vi "Write JSON Config.vi"(6 "Pretty Print?":bool, 8 "error in (no error)":errorcluster, 11 "ConvertTo_String in":refnum<class "ConvertTo_String.lvclass">) -> (0 "error out":errorcluster, 2 "JSON":string, 3 "ConvertTo_String out":refnum<class "ConvertTo_String.lvclass">)   [LabVIEW 2021, in "ConvertTo_String.lvclass"]
uses:
  ConvertTo_String.lvclass
  C:/Program Files (x86)/National Instruments/LabVIEW 2021/vi.lib/TSA/Abstract Data Classes/Abs_Types/Type/Abs_Type.lvclass
  ConvertTo_String.lvclass/ConvertTo_String.ctl
  <vilib>/JDP Science/JSONtext/Make JSON Array.vi
  <vilib>/JDP Science/JSONtext/Merge into Object.vi
  <vilib>/JDP Science/JSONtext/Make JSON Object.vi
  <vilib>/Utility/LVClass/Get LV Class Name.vi
  <vilib>/JDP Science/JSONtext/support/Format JSON Array Text.vi
  <vilib>/JDP Science/JSONtext/support/Format JSON Object.vi
  <vilib>/JDP Science/JSONtext/Get all Object Items.vi
  <vilib>/JDP Science/JSONtext/Set Multiple Object Items.vi
  Abs_Types/Value/Abs_Value.lvclass
  Abs_Types/String/Abs_String.lvclass
  Abs_Types/Type/Abs_Type.lvclass
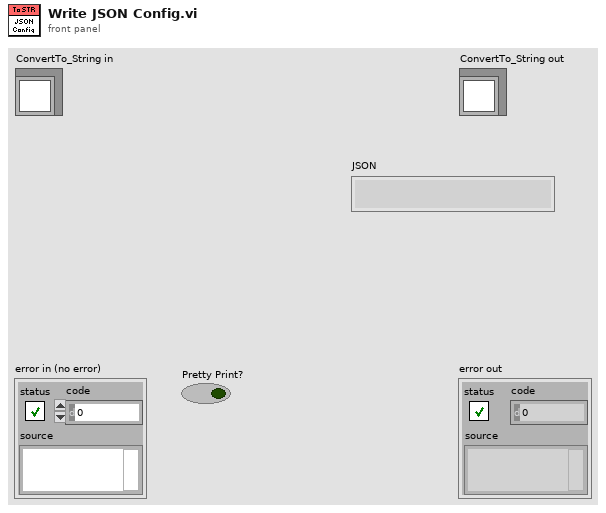
[diagram p1: front panel]
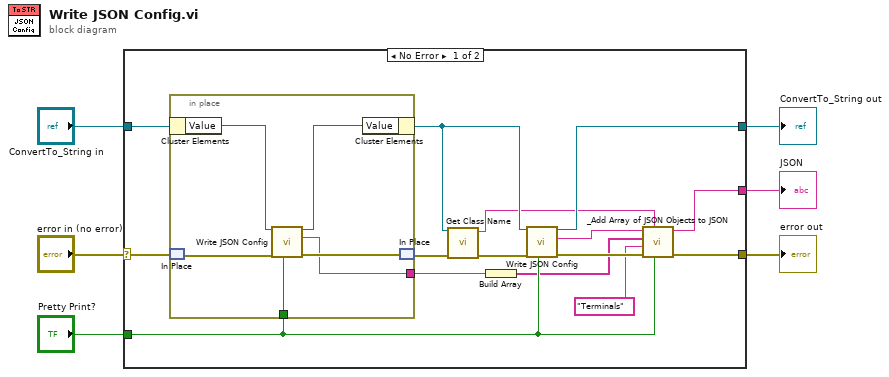
[diagram p0: block diagram]
diagram:
  n1 = case shown="No Error" "error in (no error)" {
    selector: "error in (no error)" -> [w17 w29]
    tunnel: "ConvertTo_String in" -> [w21 w28]
    tunnel: [w20 w28] -> w3
    tunnel: [w13 _] -> w2
    tunnel: [w12 w29] -> w1
    tunnel: "Pretty Print?" -> [w11 _]
    frame No Error {
      n2 = in-place {
        in-place-border: w11 -> [w26]
        in-place-border: [w24] -> w19
        n3 = in-place-cluster #1(w21) -> ("Value"=w23:refnum<class "Abs_Value.lvclass">)
        n4 = in-place-match #2(w17) -> (w27:errorcluster)
        n5 = call-dynamic "Write JSON Config.vi"("Pretty Print?"=w26, "error in (no error)"=w27, "Abs_Type in"=w23) -> ("error out"=w25:errorcluster, "JSON"=w24:string, "Abs_Type out"=w22:refnum<class "Abs_Value.lvclass">)  [unwired: 6 in]
        n6 = in-place-cluster #1("Value"=w22) -> (w15:refnum<class "ConvertTo_String.lvclass">)
        n7 = in-place-match #2(w25) -> (w18:errorcluster)
      }
      n8 = call "Get Class Name.vi"("error in (no error)"=w18, "Abs_Type in"=w15) -> ("error out"=w16:errorcluster, "class name"=w10:string)  [unwired: 8 in]
      n9 = Build Array(w19) -> (w8:string[])
      n10 = call-parent "Write JSON Config.vi"("Pretty Print?"=w11, "error in (no error)"=w16, "Abs_Type in"=w15) -> ("error out"=w14:errorcluster, "JSON"=w9:string, "Abs_Type out"=w20:refnum<class "ConvertTo_String.lvclass">)  [unwired: 6 in]
      n11 = call "_Add Array of JSON Objects to JSON.vi"("Pretty Print?"=w11, "JSON Object Name"=w10, "error in (no error)"=w14, "JSON Array Name"="Terminals", "JSON Objects"=w8, "JSON"=w9) -> ("error out"=w12:errorcluster, "<JSON>"=w13:string)  [unwired: 4 in]
    }
    frame Error {
    }
  }
  "error out" <- w1
  "ConvertTo_String out" <- w3
  "JSON" <- w2
